vi "CLD 5 Parse Config Data File.vi"(8 "error in (no error)":errorcluster, 10 "Array In":T1[][](array[typedef]), 11 "Get/Set":enum16{"Get", "Set"}(ring)) -> (0 "error out":errorcluster, 3 "Array Out":T1[][](array[typedef]))   [LabVIEW 2009]
doc: "CLD 5 exercise"
uses:
  CLD 5 Data Cluster.ctl
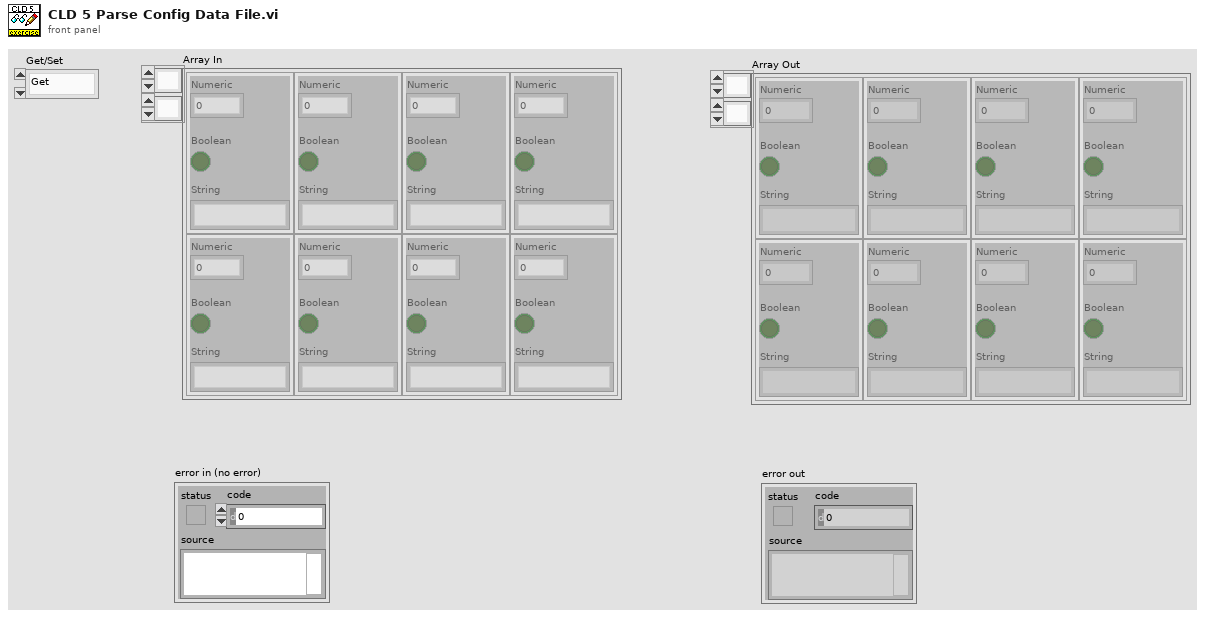
[diagram p1: front panel]
types:
  T1 = typedef "CLD 5 Data Cluster.ctl" = cluster{"Numeric":dbl, "Boolean":bool, "String":string}
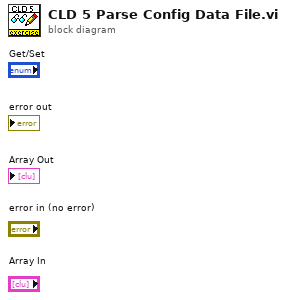
[diagram p0: block diagram]
diagram:
